vi "AdvanceToNextProjectItem.vi"(8 "error in (no error)":errorcluster, 11 "BuildManager in":refnum<class "BuildManager.lvclass">) -> (0 "error out":errorcluster, 3 "BuildManager out":refnum<class "BuildManager.lvclass">)   [LabVIEW 2020, in "SolutionBuilder.lvlib" / "BuildManager.lvclass"]
uses:
  BuildManager.lvclass
  <vilib>/Utility/miscctls.llb/LVReplaceWithSaveOptionEnum.ctl
  BuildManager.lvclass/BuildManager.ctl
  ProjectItem/ProjectItem.lvclass
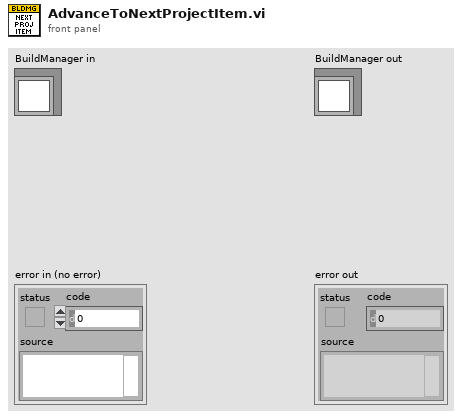
[diagram p1: front panel]
types:
  T1 = typedef "LVReplaceWithSaveOptionEnum.ctl" = enum16{"Save All Without Prompts", "Save All With Prompts", "Do Not Save (Retain In Memory)"}
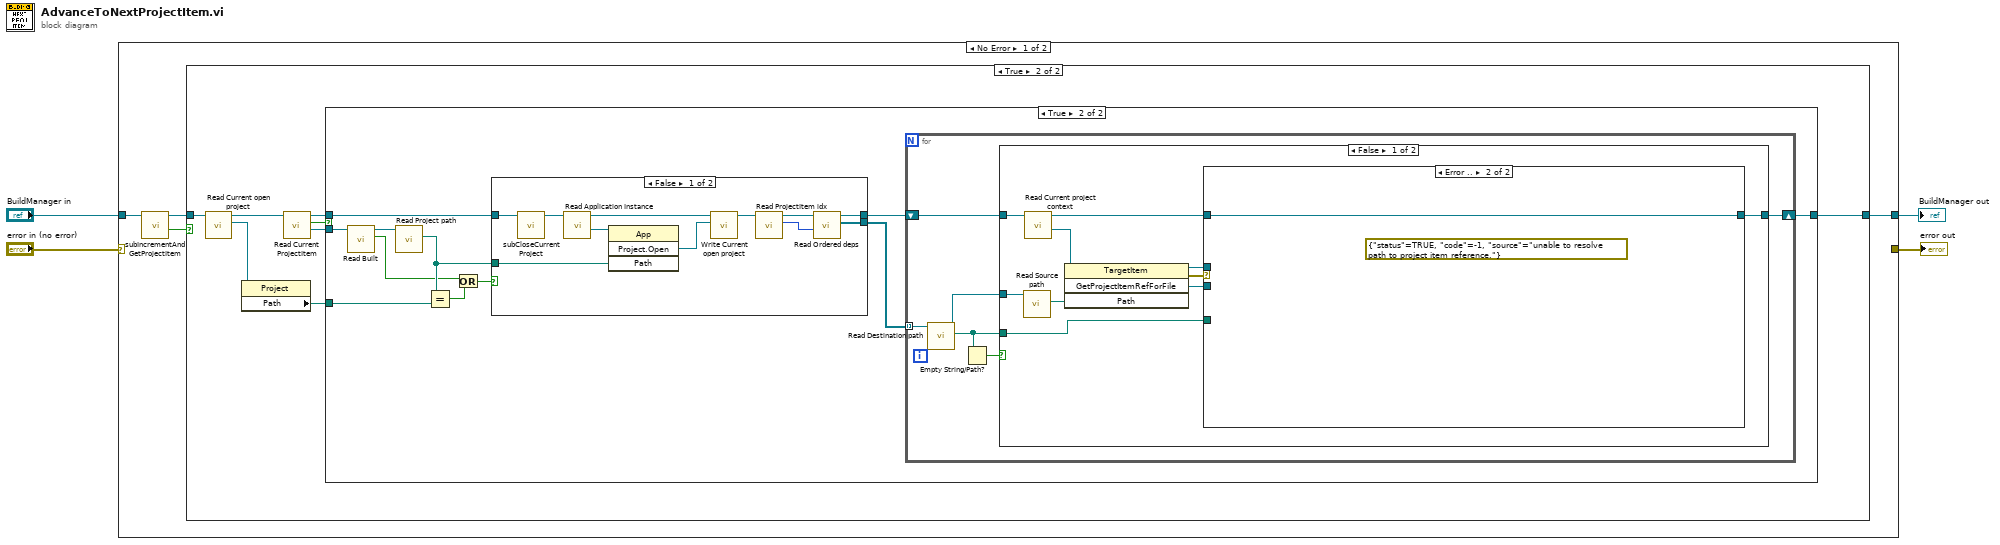
[diagram p0: block diagram]
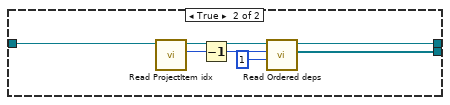
[diagram p4: hidden frame]
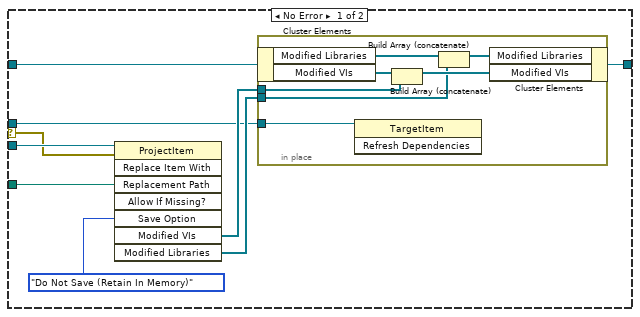
[diagram p5: hidden frame]
diagram:
  n1 = case shown="No Error" "error in (no error)" {
    selector: "error in (no error)" -> [_ w82]
    tunnel: [w8 w83] -> w4
    tunnel: "BuildManager in" -> [w7 w83]
    tunnel: [_ w82] -> w1
    frame No Error {
      n2 = call "subIncrementAndGetProjectItem.vi"("BuildManager in"=w7) -> ("Valid"=w5:bool, "BuildManager out"=w6:refnum<class "BuildManager.lvclass">)  [unwired: 8 in, 1 out]
      n3 = case shown="True" w5 {
        tunnel: [w9 w16] -> w8
        tunnel: w6 -> [w9 w14]
        frame False {
        }
        frame True {
          n4 = call-dynamic "Read Current open project.vi"("BuildManager in"=w14) -> ("Current open project"=w15:refnum<vi>, "BuildManager out"=w13:refnum<class "BuildManager.lvclass">)  [unwired: 9 in]
          n5 = property class="Project"(reference=w15) -> ("Path"=w17:path)  [unwired: 1 in, 2 out]
          n6 = call-dynamic "Read Current ProjectItem.vi"("BuildManager in"=w13) -> ("Current ProjectItem"=w10:refnum<class "ProjectItem.lvclass">, "Valid"=w11:bool, "BuildManager out"=w12:refnum<class "BuildManager.lvclass">)  [unwired: 8 in]
          n7 = case shown="True" w11 {
            tunnel: w17 -> [_ w29]
            tunnel: [w18 w27] -> w16
            tunnel: w12 -> [w18 w26]
            tunnel: w10 -> [_ w22]
            frame False {
            }
            frame True {
              n8 = call-dynamic "Read Built.vi"("ProjectItem in"=w22) -> ("Built"=w20:bool, "ProjectItem out"=w23:refnum<class "ProjectItem.lvclass">)  [unwired: 9 in]
              n9 = call-dynamic "Read Project path.vi"("ProjectItem in"=w23) -> ("Project path"=w28:path)  [unwired: 9 in, 1 out]
              n10 = Equal?(x=w28, y=w29) -> (x = y?=w21:bool)
              n11 = Or(x=w20, y=w21) -> (x .or. y?=w19:bool)
              n12 = case shown="False" w19 {
                tunnel: w26 -> [w40 w47]
                tunnel: [w32 w44] -> w24
                tunnel: w28 -> [w39 _]
                tunnel: [w30 w41] -> w25
                frame False {
                  n13 = call "subCloseCurrentProject.vi"("BuildManager in"=w40) -> ("BuildManager out"=w38:refnum<class "BuildManager.lvclass">)  [unwired: 9 in, 1 out]
                  n14 = call-dynamic "Read Application Instance.vi"("BuildManager in"=w38) -> ("Application Instance"=w37:refnum<vi>, "BuildManager out"=w36:refnum<class "BuildManager.lvclass">)  [unwired: 9 in]
                  n15 = invoke class="App" method="Project.Open"(reference=w37, "Path"=w39) -> ("Project:Open"=w35:refnum<vi>)  [unwired: 2 in, 3 out]
                  n16 = call-dynamic "Write Current open project.vi"("Current open project"=w35, "BuildManager in"=w36) -> ("BuildManager out"=w34:refnum<class "BuildManager.lvclass">)  [unwired: 9 in]
                  n17 = call-dynamic "Read ProjectItem idx.vi"("BuildManager in"=w34) -> ("ProjectItem idx"=w31:i32, "BuildManager out"=w33:refnum<class "BuildManager.lvclass">)  [unwired: 9 in]
                  n18 = call-dynamic "Read Ordered deps.vi"("length (-1)"=w31, "BuildManager in"=w33) -> ("Ordered deps"=w30:refnum<class "ProjectItem.lvclass">[], "BuildManager out"=w32:refnum<class "BuildManager.lvclass">)  [unwired: 8 in]
                }
                frame True {
                  n19 = call-dynamic "Read ProjectItem idx.vi"("BuildManager in"=w47) -> ("ProjectItem idx"=w46:i32, "BuildManager out"=w45:refnum<class "BuildManager.lvclass">)  [unwired: 9 in]
                  n20 = Decrement(x=w46) -> (x-1=w43:i32)
                  n21 = call-dynamic "Read Ordered deps.vi"("length (-1)"=1, "index"=w43, "BuildManager in"=w45) -> ("Ordered deps"=w41:refnum<class "ProjectItem.lvclass">[], "BuildManager out"=w44:refnum<class "BuildManager.lvclass">)  [unwired: 7 in]
                }
              }
              n22 = for {
                shift-right: [w48] -> w27
                shift-left: w24 -> [w49]
                tunnel: w25 -> [w53] mode=indexing
                n23 = call-dynamic "Read Destination path.vi"("ProjectItem in"=w53) -> ("Destination path"=w51:path, "ProjectItem out"=w52:refnum<class "ProjectItem.lvclass">)  [unwired: 9 in]
                n24 = Empty String/Path?(string/path=w51) -> (empty?=w50:bool)
                n25 = case shown="False" w50 {
                  tunnel: w52 -> [w61 _]
                  tunnel: w51 -> [w60 _]
                  tunnel: w49 -> [w56 w81]
                  tunnel: [w58 w81] -> w48
                  frame False {
                    n26 = call-dynamic "Read Source path.vi"("ProjectItem in"=w61) -> ("Source path"=w63:path)  [unwired: 9 in, 1 out]
                    n27 = call-dynamic "Read Current project context.vi"("BuildManager in"=w56) -> ("Project context"=w54:refnum<vi>, "BuildManager out"=w55:refnum<class "BuildManager.lvclass">)  [unwired: 9 in]
                    n28 = invoke class="TargetItem" method="GetProjectItemRefForFile"(reference=w54, "Path"=w63) -> (reference out=w57:refnum<vi>, error out=w59:errorcluster, "GetProjectItemRefForFile"=w62:refnum<vi>)  [unwired: 2 in, 1 out]
                    n29 = case shown="Error .." w59 {
                      selector: w59 -> [w65 _]
                      tunnel: w62 -> [w71 _]
                      tunnel: w60 -> [w70 _]
                      tunnel: w55 -> [w69 w80]
                      tunnel: [w66 w80] -> w58
                      tunnel: w57 -> [w64 _]
                      frame No Error {
                        n30 = invoke class="ProjectItem" method="Replace Item With"(reference=w71, error in=w65, "Replacement Path"=w70, "Save Option"=LVReplaceWithSaveOptionEnum."Do Not Save (Retain In Memory)") -> ("Modified VIs"=w68:refnum<vi>[], "Modified Libraries"=w67:refnum<vi>[])  [unwired: 4 in, 6 out]
                        n31 = in-place {
                          in-place-border: w68 -> [w78]
                          in-place-border: w67 -> [w75]
                          in-place-border: w64 -> [w73]
                          n32 = in-place-cluster #1(w69) -> ("Modified Libraries"=w76:refnum<vi>[], "Modified VIs"=w79:refnum<vi>[])
                          n33 = invoke class="TargetItem" method="Refresh Dependencies"(reference=w73) -> ()  [unwired: 2 in, 3 out]
                          n34 = Build Array (concatenate)(w79, w78) -> (w77:refnum<vi>[])
                          n35 = Build Array (concatenate)(w76, w75) -> (w74:refnum<vi>[])
                          n36 = in-place-cluster #1("Modified Libraries"=w74, "Modified VIs"=w77) -> (w66:refnum<class "BuildManager.lvclass">)
                        }
                      }
                      frame Error {
                        (unwired) errorcluster {"status"=TRUE, "code"=-1, "source"="unable to resolve path to project item reference."} ("t")
                      }
                    }
                  }
                  frame True {
                  }
                }
              }
            }
          }
        }
      }
    }
    frame Error {
    }
  }
  "error out" <- w1
  "BuildManager out" <- w4
